vi "RightShiftX.vi"(8 "Shift":i32, 9 "Data":i32 format="%.0x") -> (1 "Shifted Data":i32 format="%.0x")   [LabVIEW 2010]
doc: "This VI right shifts the input data by X and preserves the sign of the number."
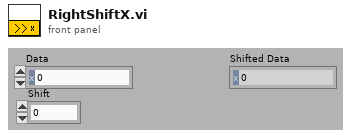
[diagram p1: front panel]
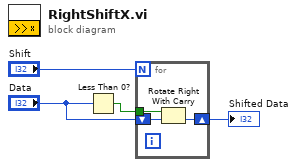
[diagram p0: block diagram]
diagram:
  n1 = Less Than 0?(x="Data") -> (x < 0?=w3:bool)
  n2 = for {
    N: "Shift" -> [_]
    tunnel: w3 -> [w6]
    shift-right: [w5] -> w1
    shift-left: "Data" -> [w7]
    n3 = Rotate Right With Carry(2:w7, 3:w6) -> (0:w5:i32)  [unwired: 1 out]
  }
  "Shifted Data" <- w1
